vi "Note Popup.vi"(10 "SR Number":i32) -> ()   [LabVIEW 2018]
uses:
  <vilib>/Utility/miscctls.llb/LVPositionTypeDef.ctl
panel:
  in  "Cancel Button":bool
  in  "Save Button":bool
  in  "Notes":string
  out "Error Out":errorcluster
  in  "Error In":errorcluster
  out "Help Text":string
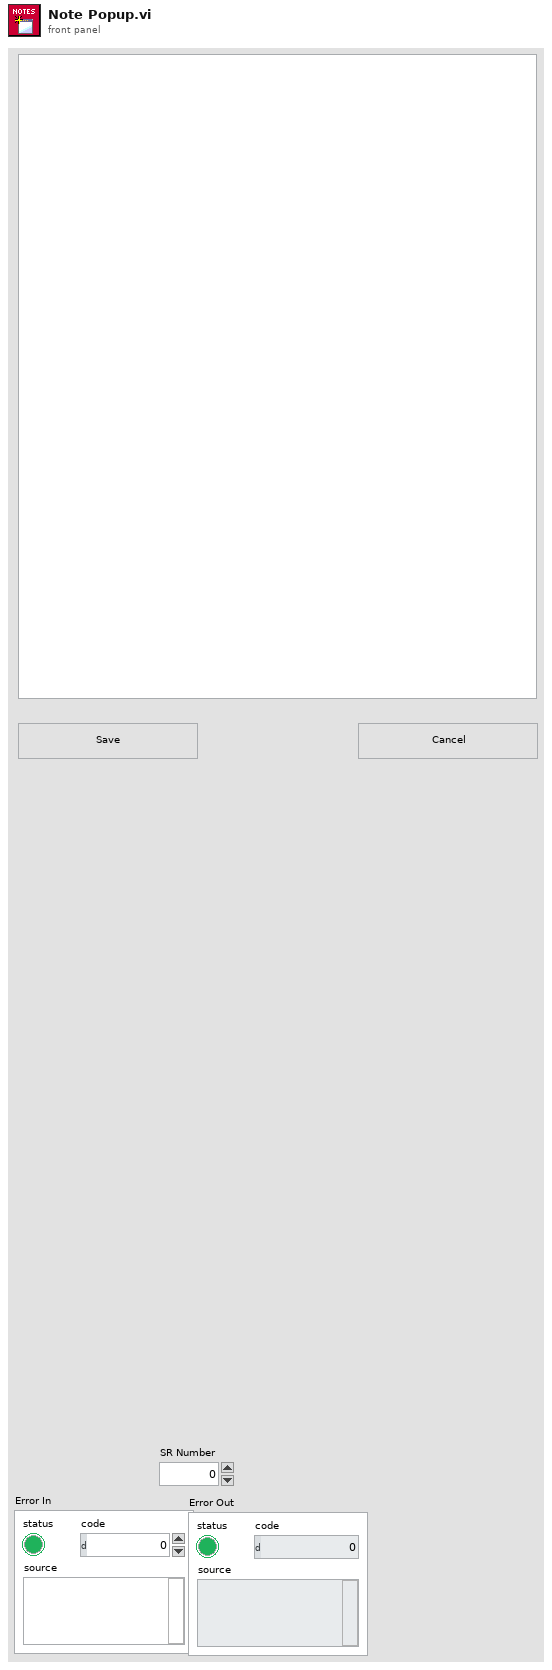
[diagram p1: front panel]
types:
  T1 = typedef "LVPositionTypeDef.ctl" = cluster{"Left":i32, "Top":i32}
  T2 = enum16{"Always On", "Always Off", "Off While Running"}
  T3 = enum16{"Left Button", "Center Button", "Right Button", "Window Close"}
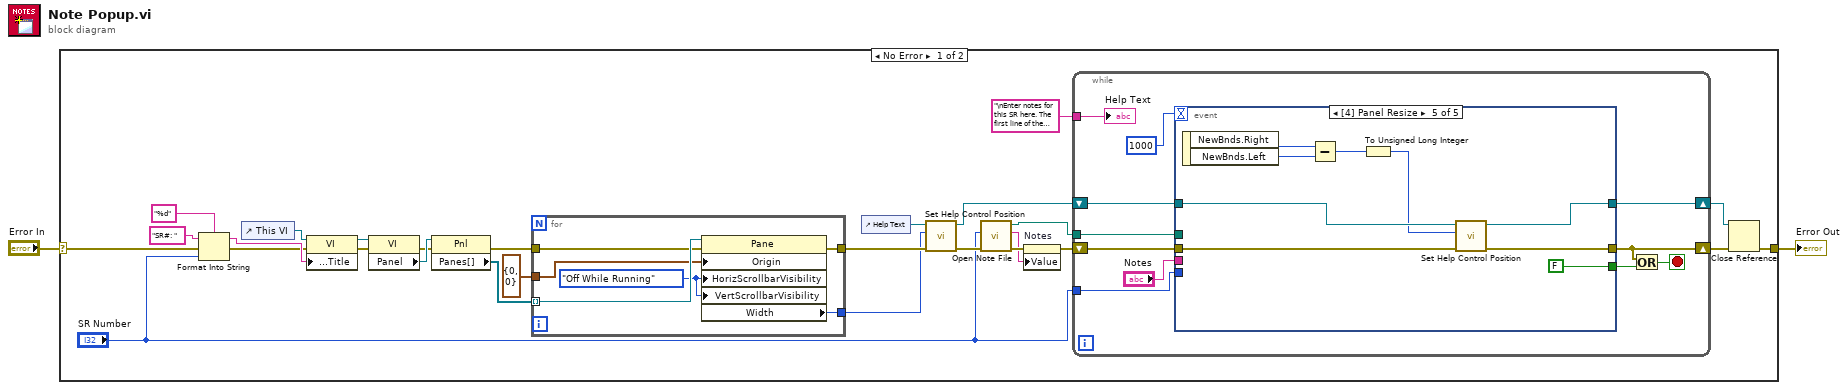
[diagram p0: block diagram]
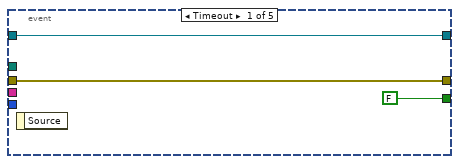
[diagram p2: hidden frame]
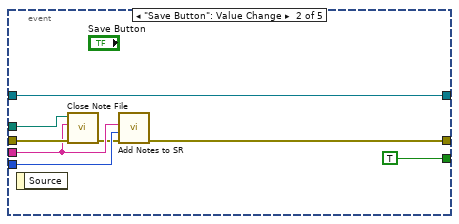
[diagram p3: hidden frame]
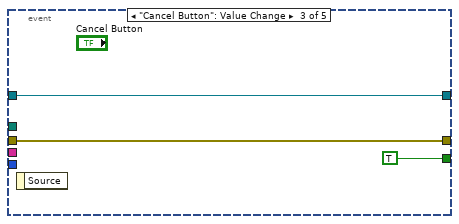
[diagram p4: hidden frame]
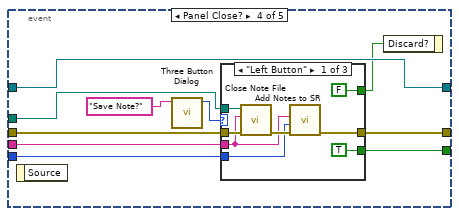
[diagram p5: hidden frame]
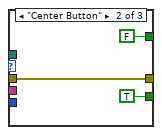
[diagram p6: hidden frame]
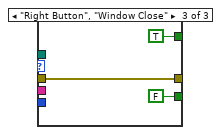
[diagram p7: hidden frame]
diagram:
  n1 = case shown="No Error" "Error In" {
    selector: "Error In" -> [w7 w94]
    tunnel: [w6 w94] -> w2
    frame No Error {
      n2 = Format Into String(format string="%d", initial string="SR#: ", error in=w7, "SR Number") -> (resulting string=w26:string, error out=w25:errorcluster)
      n3 = control-ref of="This VI"() -> (w28:refnum<vi>)
      n4 = property class="VI"(reference=w28, error in=w25, "Front Panel.Title"=w26) -> (reference out=w23:refnum<vi>, error out=w22:errorcluster)
      n5 = property class="VI"(reference=w23, error in=w22) -> (error out=w20:errorcluster, "Panel"=w21:refnum<vi>)  [unwired: 1 out]
      n6 = property class="Pnl"(reference=w21, error in=w20) -> (error out=w18:errorcluster, "Panes[]"=w14:refnum<vi>[])  [unwired: 1 out]
      n7 = for {
        tunnel: w14 -> [w35] mode=indexing
        tunnel: T1 {"Left"=0, "Top"=0} ("Position") -> [w34]
        tunnel: w18 -> [w33]
        tunnel: [w32] -> w11
        tunnel: [w30] -> w10
        w31 = T2."Off While Running" ("Horizontal Scrollbar Visibility")
        n8 = property class="Pane"(reference=w35, error in=w33, "Origin"=w34, "HorizScrollbarVisibility"=w31, "VertScrollbarVisibility"=w31) -> (error out=w32:errorcluster, "Width"=w30:u32)  [unwired: 1 out]
      }
      n9 = control-ref of="Help Text"() -> (w12:refnum<vi>)
      n10 = call "Set Help Control Position.vi"("error in (no error)"=w11, "Width"=w10, "String in"=w12) -> ("error out"=w8:errorcluster, "String out"=w9:refnum<vi>)  [unwired: 7 in]
      n11 = call "Open Note File.vi"("Error In"=w8, "SR Number"="SR Number") -> ("Error Out"=w17:errorcluster, "Notes"=w15:string, "file path"=w29:path)  [unwired: 7 in]
      n12 = property on="Notes" class="Str"(error in=w17, "Value"=w15) -> (error out=w16:errorcluster)  [unwired: 1 in, 1 out]
      n13 = while {
        tunnel: w29 -> [w43]
        shift-right: [w40] -> w4
        shift-left: w16 -> [w45]
        tunnel: "\nEnter notes for this SR here. The first line of the entered text will be displayed on the front panel." ("Help Text") -> [w39]
        shift-right: [w37] -> w5
        shift-left: w9 -> [w38]
        tunnel: "SR Number" -> [w36]
        stop <- w42 stop-if-true
        n14 = event shown="[4] Panel Resize" {
          selector: _ -> [_ _ _ _ _]
          dyn-events: _ -> [_ _ _ _ _]
          timeout: 1000 -> [_ _ _ _ _]
          tunnel: [FALSE TRUE TRUE w69 FALSE] -> w41
          tunnel: w45 -> [w48 w56 w59 w68 w90]
          tunnel: [w48 w50 w59 w67 w89] -> w40
          tunnel: "Notes" -> [_ w53 _ w66 _]
          tunnel: w43 -> [_ w55 _ w63 _]
          tunnel: w38 -> [w47 w54 w58 w65 w87]
          tunnel: [w47 w54 w58 w65 w88] -> w37
          tunnel: w36 -> [_ w52 _ w62 _]
          event Timeout {
            n15 = event-data() -> ()  [unwired: 1 in, 1 out]
          }
          event "Save Button": Value Change {
            n16 = event-data() -> ()  [unwired: 1 in, 1 out]
            n17 = call "Close Note File.vi"("Error In"=w56, "Notes"=w53, "file path"=w55) -> ("Error Out"=w51:errorcluster)  [unwired: 8 in]
            n18 = call "Add Notes to SR.vi"("Error In"=w51, "SR Number"=w52, "Note to Add"=w53) -> ("Error Out"=w50:errorcluster)  [unwired: 8 in]
          }
          event "Cancel Button": Value Change {
            n19 = event-data() -> ()  [unwired: 1 in, 1 out]
          }
          event Panel Close? {
            n20 = event-data() -> ()  [unwired: 1 in, 1 out]
            n21 = call <vilib>:"Three Button Dialog.vi"("message"="Save Note?") -> ("Which Button?"=w64:T3)  [unwired: 10 in]
            n22 = case shown="\"Left Button\"" w64 {
              tunnel: [FALSE ("Discard?") FALSE ("Discard?") TRUE ("Discard?")] -> w61
              tunnel: [TRUE TRUE FALSE] -> w69
              tunnel: w68 -> [w76 w79 w82]
              tunnel: [w74 w79 w82] -> w67
              tunnel: w66 -> [w71 _ _]
              tunnel: w63 -> [w75 _ _]
              tunnel: w62 -> [w72 _ _]
              frame "Left Button" {
                n23 = call "Close Note File.vi"("Error In"=w76, "Notes"=w71, "file path"=w75) -> ("Error Out"=w73:errorcluster)  [unwired: 8 in]
                n24 = call "Add Notes to SR.vi"("Error In"=w73, "SR Number"=w72, "Note to Add"=w71) -> ("Error Out"=w74:errorcluster)  [unwired: 8 in]
              }
              frame "Center Button" {
              }
              frame "Right Button", "Window Close" {
              }
            }
            n25 = event-data("Discard?"=w61) -> ()  [unwired: 1 in, 1 out]
          }
          event Panel Resize {
            n26 = event-data() -> ("NewBnds.Right"=w92:i16, "NewBnds.Left"=w91:i16)  [unwired: 1 in]
            n27 = Subtract(x=w92, y=w91) -> (x-y=w86:i16)
            n28 = To Unsigned Long Integer(number=w86) -> (unsigned 32bit integer=w85:u32)
            n29 = call "Set Help Control Position.vi"("error in (no error)"=w90, "Width"=w85, "String in"=w87) -> ("error out"=w89:errorcluster, "String out"=w88:refnum<vi>)  [unwired: 7 in]
          }
        }
        n30 = Or(x=w40, y=w41) -> (x .or. y?=w42:bool)
        "Help Text" <- w39
      }
      n31 = Close Reference(reference=w5, error in (no error)=w4) -> (error out=w6:errorcluster)
    }
    frame Error {
    }
  }
  "Error Out" <- w2
